vi "Timestamp to DATE-DT Byte Stream.vi"(8 "error in (no error)":errorcluster, 10 "Value":timestamp) -> (0 "error out":errorcluster, 2 "Byte Stream":u8[](array[numeric]))   [LabVIEW 2018, in "TwinCAT ADS.lvclass"]
uses:
  TwinCAT ADS.lvclass
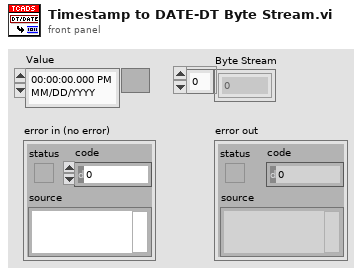
[diagram p1: front panel]
types:
  T1 = enum16{"big-endian, network order", "native, host order", "little-endian"}
  T2 = typedef "LVDateTimeRec.ctl" = cluster{"fractional second":dbl, "second":i32, "minute":i32, "hour":i32, "day of month":i32, "month":i32, "year":i32, "day of week":i32, "day of year":i32, "DST":i32}
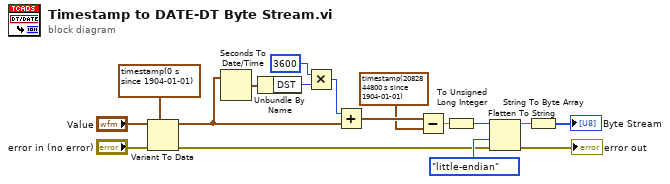
[diagram p0: block diagram]
diagram:
  n1 = Variant To Data(error in="error in (no error)", type=timestamp(0 s since 1904-01-01), Variant="Value") -> (data=w12:timestamp, error out=w2:errorcluster)
  n2 = Seconds To Date/Time(time stamp (now)=w12) -> (date time rec=w10:T2)  [unwired: 1 in]
  n3 = Unbundle By Name(w10) -> ("DST"=w7:i32)
  n4 = Multiply(x=3600, y=w7) -> (x*y=w8:i32)
  n5 = Add(x=w8, y=w12) -> (x+y=w11:timestamp)
  n6 = Subtract(x=w11, y=timestamp(2082844800 s since 1904-01-01) ("time stamp")) -> (x-y=w1:dbl)
  n7 = To Unsigned Long Integer(number=w1) -> (unsigned 32bit integer=w17:u32)
  n8 = Flatten To String(anything=w17, byte order (0:big-endian, network order)=T1."little-endian", error in (no error)=w2) -> (data string=w15:string, error out=→"error out":errorcluster)  [unwired: 1 in, 1 out]
  n9 = String To Byte Array(string=w15) -> (unsigned byte array=→"Byte Stream":u8[])
